vi "Put Data.vi"(8 "error in (no error)":errorcluster, 9 "Path in":string, 10 "Data":refnum<class "Data.lvclass">, 11 "Connection in":refnum<class "Connection.lvclass">) -> (0 "error out":errorcluster, 3 "Connection out":refnum<class "Connection.lvclass">)   [LabVIEW 2015, in "MDSplus.lvlib" / "Connection.lvclass"]
uses:
  <userlib>/MDSplus/Classes/Connection_Class/Connection.lvclass
  <userlib>/MDSplus/Classes/Data_Class/Data.lvclass
  <userlib>/MDSplus/Classes/Connection_Class/Connection.lvclass/Connection.ctl
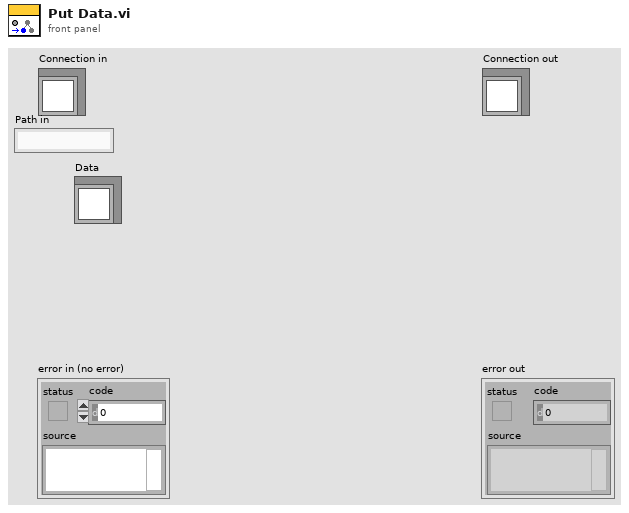
[diagram p1: front panel]
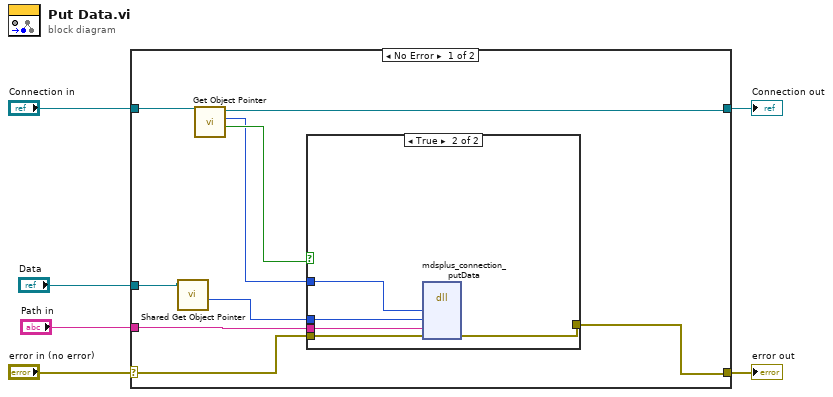
[diagram p0: block diagram]
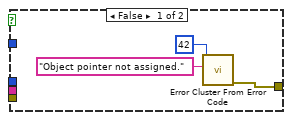
[diagram p2: hidden frame]
diagram:
  n1 = case shown="No Error" "error in (no error)" {
    selector: "error in (no error)" -> [w9 w25]
    tunnel: [w8 w25] -> w5
    tunnel: [w14 w24] -> w3
    tunnel: "Connection in" -> [w15 w24]
    tunnel: "Data" -> [w12 _]
    tunnel: "Path in" -> [w7 _]
    frame No Error {
      n2 = call <userlib>:"Shared Get Object Pointer.vi"("Data in"=w12) -> ("Object Pointer"=w11:i64)  [unwired: 8 in, 2 out]
      n3 = call <userlib>:"Get Object Pointer.vi"("Connection in"=w15) -> ("Assigned object pointer?"=w13:bool, "Object Pointer"=w10:i64, "Connection out"=w14:refnum<class "Connection.lvclass">)  [unwired: 7 in, 1 out]
      n4 = case shown="True" w13 {
        tunnel: [w16 w20] -> w8
        tunnel: w11 -> [_ w23]
        tunnel: w10 -> [_ w22]
        tunnel: w9 -> [_ w21]
        tunnel: w7 -> [_ w19]
        frame False {
          n5 = call <vilib>:"Error Cluster From Error Code.vi"("error message (\"\")"="Object pointer not assigned." ("error message (\"\")"), "error code (0)"=42) -> ("error out"=w16:errorcluster)  [unwired: 7 in]
        }
        frame True {
          n6 = dll-call lib="MDSobjectsLVShr" fn="mdsplus_connection_putData"("lvConnection"=w22, "lvDataPtrIn"=w23, "pathIn"=w19, "error"=w21) -> ("error"=w20:errorcluster)  [unwired: 7 in, 2 out]
        }
      }
    }
    frame Error {
    }
  }
  "error out" <- w5
  "Connection out" <- w3
